vi "16-sub-calc-num-dig.vi"(4 "base in":u64, 5 "exponent in":u64) -> (1 "Number of Digits":i32)   [LabVIEW 2021]
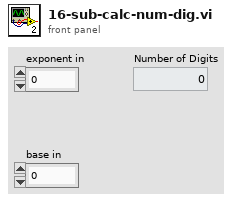
[diagram p1: front panel]
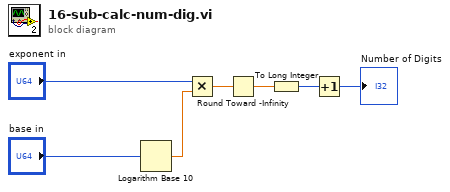
[diagram p0: block diagram]
diagram:
  n1 = Logarithm Base 10(1:"base in") -> (0:w1:dbl)
  n2 = Multiply(x="exponent in", y=w1) -> (x*y=w2:dbl)
  n3 = Round Toward -Infinity(1:w2) -> (0:w3:dbl)
  n4 = To Long Integer(number=w3) -> (32bit integer=w4:i32)
  n5 = Increment(x=w4) -> (x+1=→"Number of Digits":i32)
